vi "Format Client Request (Auto-Increment).vi"(8 "error in (no error)":errorcluster, 9 "initial string":string, 10 "JSON in":refnum<class "JSON Null.lvclass">, 11 "method":string) -> (0 "error out":errorcluster, 2 "Request String":string)   [LabVIEW 2015, in "JSONRPC Server.lvclass"]
uses:
  JSONRPC Server.lvclass
  <vilib>/National Instruments/JSON Support for LabVIEW/JSON Data Classes/JSON Datatype/JSON Null.lvclass
  <vilib>/National Instruments/JSON Support for LabVIEW/JSON Data Classes/JSON Object/Insert Key Value Pair (Single String).vi
  <vilib>/National Instruments/JSON Support for LabVIEW/JSON Data Classes/JSON Object/JSON Object.lvclass
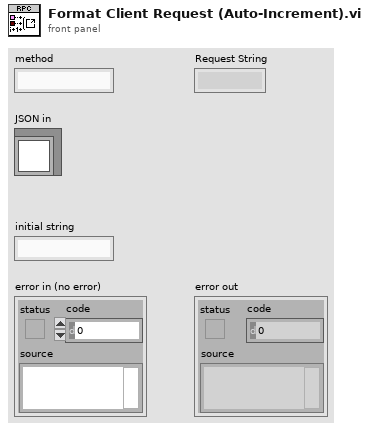
[diagram p1: front panel]
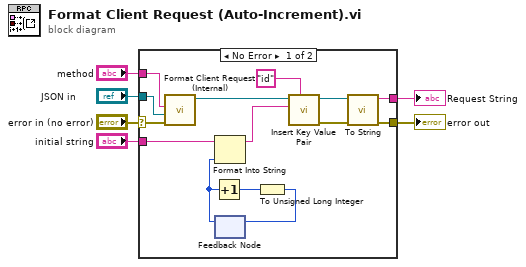
[diagram p0: block diagram]
diagram:
  n1 = case shown="No Error" "error in (no error)" {
    selector: "error in (no error)" -> [w20 w21]
    tunnel: [w7 w21] -> w5
    tunnel: "JSON in" -> [w18 _]
    tunnel: "method" -> [w19 _]
    tunnel: "initial string" -> [w17 _]
    tunnel: [w8 _] -> w1
    frame No Error {
      n2 = call "Format Client Request (Internal).vi"("error in (no error)"=w20, "params"=w18, "method"=w19) -> ("JSON Object out"=w11:refnum<class "JSON Object.lvclass">)  [unwired: 7 in, 1 out]
      n3 = feedback #1() -> (w16:u32)  [unwired: 1 in]
      n4 = Increment(x=w16) -> (x+1=w15:u32)
      n5 = Format Into String(initial string=w17, w16) -> (resulting string=w10:string)  [unwired: 2 in, 1 out]
      n6 = To Unsigned Long Integer(number=w15) -> (unsigned 32bit integer=w14:u32)
      n7 = feedback-in #1(w14) -> ()
      n8 = call-poly <vilib>:"Insert Key Value Pair.vi"("key"="id" ("Name"), "value"=w10, "JSON Object in"=w11) -> ("error out"=w12:errorcluster, "JSON Object out"=w13:refnum<class "JSON Object.lvclass">)  [unwired: 6 in, 1 out]
      n9 = call-dynamic "To String.vi"("error in (no error)"=w12, "JSON Object in"=w13) -> ("error out"=w7:errorcluster, "String"=w8:string)  [unwired: 8 in]
    }
    frame Error {
    }
  }
  "error out" <- w5
  "Request String" <- w1
